vi "executeCommand.vi"(8 "error in (no error)":errorcluster, 9 "Variant":variant, 10 "Command":T1, 11 "DomeCommunicator in":refnum<class "ATDomeCommunicator.lvclass">) -> (0 "error out":errorcluster, 3 "DomeCommunicator out":refnum<class "ATDomeCommunicator.lvclass">)   [LabVIEW 2016, in "ATDomeCommunicator.lvclass"]
uses:
  ATDomeCommunicator.lvclass
  home/plotz/lsst_ts/ss_atDome/common_labview_tcpdevice/tcpDevice/tcpDevice.lvclass
  ComTypedefs/commands.ctl
  common_labview_tcpdevice/tcpDevice/tcpDevice.lvclass
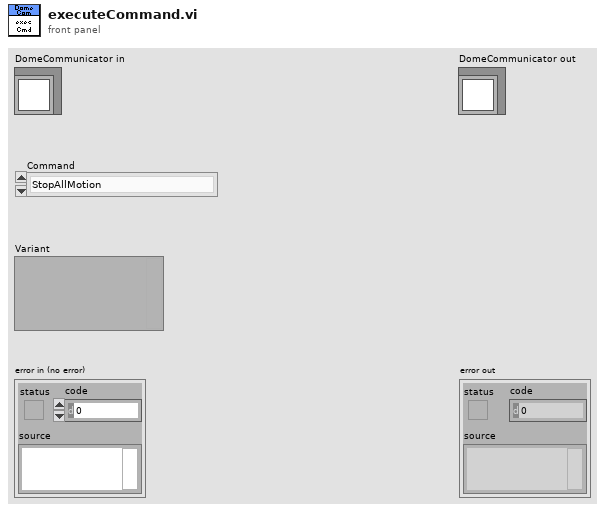
[diagram p1: front panel]
types:
  T1 = typedef "commands.ctl" = enum16{"StopAllMotion", "CloseMainDoor", "OpenMainDoor", "CloseDropoutDoor", "OpenDropoutDoor", "SynchronizedOpen", "SynchronizedClose", "AutoShutDownOn", "AutoShutDownOff", "RainOn", "RainOff", "CloudSensorOn", "CloudSensorOff", "RotateToHomePosition", "MoveToAzimuth", "SetTolerance", "DefineHomePosition", "HighSpeedThreshold", "SetCoast", "SetEncoderCountFor360", "SetWatchDogTimer", "SetReverseDirectionMotionDelay", "SaveCurrentConfiguration"}
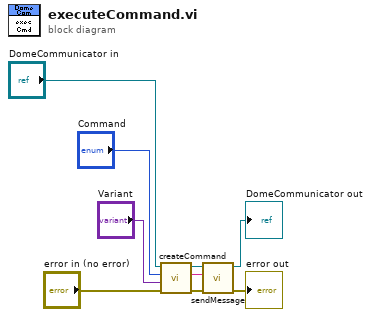
[diagram p0: block diagram]
diagram:
  n1 = call "createCommand.vi"("error in (no error)"="error in (no error)", "Variant"="Variant", "Command"="Command", "DomeCommunicator in"="DomeCommunicator in") -> ("error out"=w2:errorcluster, "CommandString"=w3:string, "DomeCommunicator out"=w5:refnum<class "ATDomeCommunicator.lvclass">)  [unwired: 5 in]
  n2 = call "sendMessage.vi"("error in (no error)"=w2, "Message"=w3, "tcpDevice in"=w5) -> ("error out"=→"error out":errorcluster, "tcpDevice out"=→"DomeCommunicator out":refnum<class "ATDomeCommunicator.lvclass">)  [unwired: 7 in]
